vi "Read XML HW Configuration File_Extra Checks.vi"(8 "error in (no error)":errorcluster, 11 "Array In":T1[](array[typedef]) {"speed" items=["Auto", "Low", "High"]; "Labels"."scheduleBuildUnit" items=["Millisecond", "Microsecond"]}) -> (0 "error out":errorcluster, 3 "Array Out":T1[](array[typedef]) {"speed" items=["Auto", "Low", "High"]; "Labels"."scheduleBuildUnit" items=["Millisecond", "Microsecond"]})   [LabVIEW 2016]
doc: "This VI performs extra checks (to what is done via the XML Deserializer with the XSD)."
uses:
  Controls/Ballard_Channel.ctl
  Controls/Ballard_Label.ctl
  Controls/Ballard_Word.ctl
  Controls/ARINCParam.ctl
  Shared/Controls and Global/TransferType.ctl
  Controls/Channel_direction.ctl
  Controls/Channel Speed.ctl
  Shared/Ballard Arinc-429 Shared.lvlib
  Ballard Arinc-429 System Explorer.lvlib
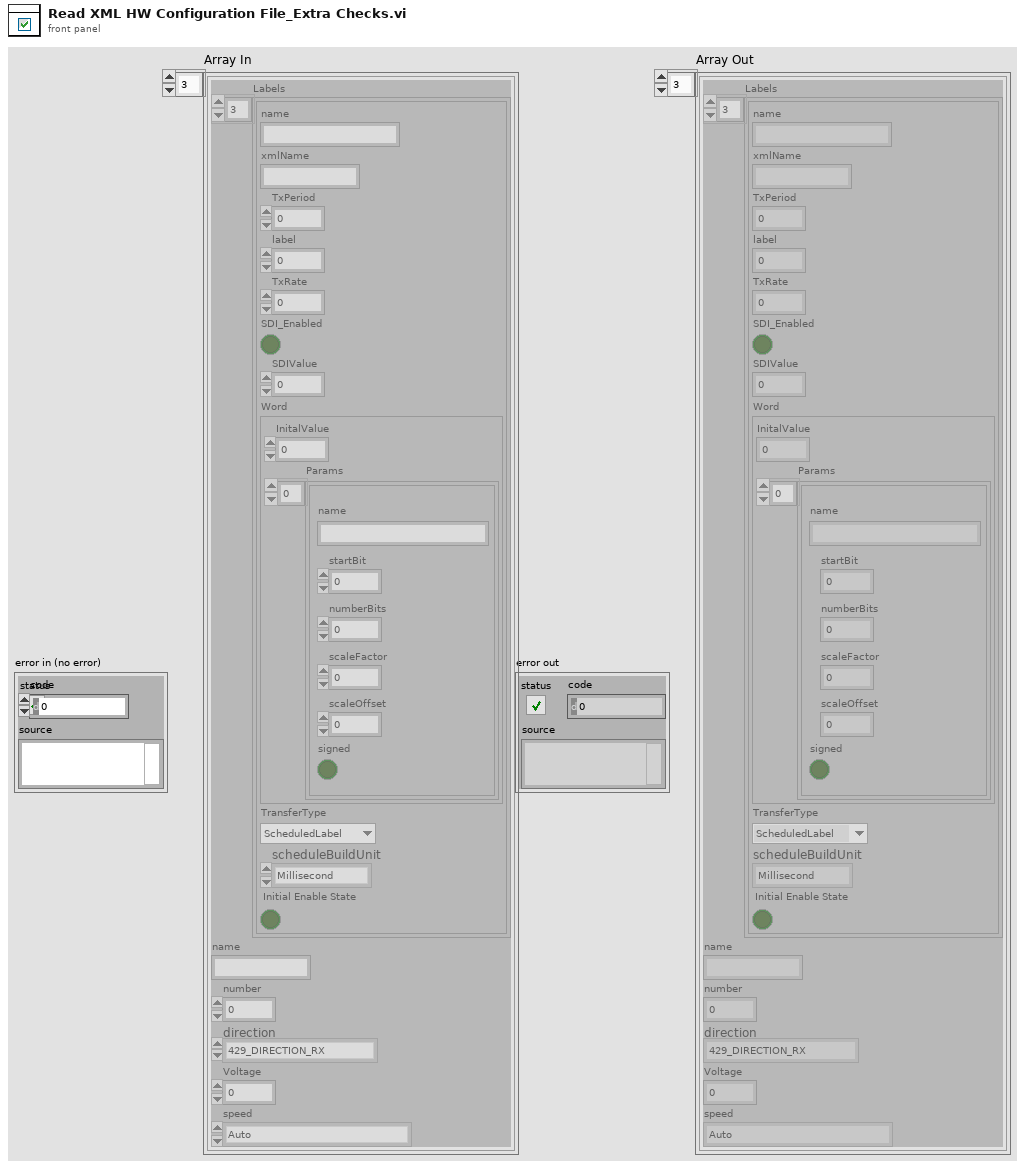
[diagram p1: front panel]
types:
  T1 = typedef "Ballard Arinc-429 System Explorer.lvlib/Ballard_Channel.ctl" = cluster{"Labels":T2[], "name":string, "number":u8, "direction":T6, "Voltage":dbl, "speed":T7}
  T2 = typedef "Ballard Arinc-429 System Explorer.lvlib/Ballard_Label.ctl" = cluster{"name":string, "xmlName":string, "TxPeriod":u32, "label":u32, "TxRate":dbl, "SDI_Enabled":bool, "SDIValue":u8, "Word":T3, "TransferType":T5, "scheduleBuildUnit":i32, "Initial Enable State":bool}
  T3 = typedef "Ballard Arinc-429 System Explorer.lvlib/Ballard_Word.ctl" = cluster{"InitalValue":u32, "Params":T4[]}
  T4 = typedef "Ballard Arinc-429 System Explorer.lvlib/ARINCParam.ctl" = cluster{"name":string, "startBit":i32, "numberBits":i32, "scaleFactor":dbl, "scaleOffset":dbl, "signed":bool}
  T5 = typedef "Ballard Arinc-429 Shared.lvlib/TransferType.ctl" = enum16{"ScheduledLabel", "Acyclic", "Block", "Strobe"}
  T6 = typedef "Ballard Arinc-429 System Explorer.lvlib/Channel_direction.ctl" = enum16{"429_DIRECTION_RX", "429_DIRECTION_TX"}
  T7 = typedef "Ballard Arinc-429 System Explorer.lvlib/Channel Speed.ctl" = i32
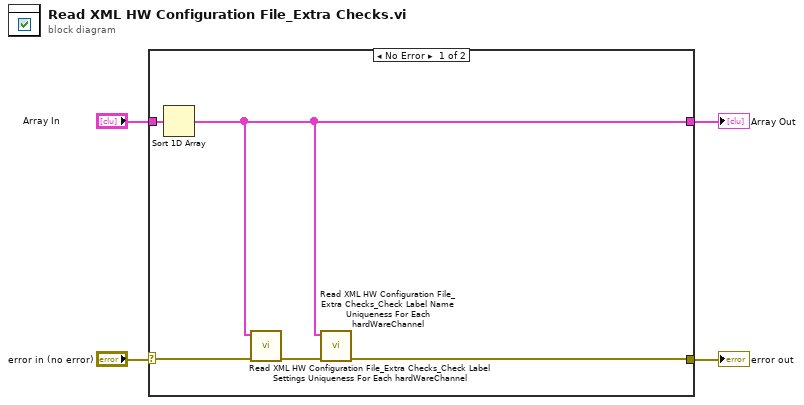
[diagram p0: block diagram]
diagram:
  n1 = case shown="No Error" "error in (no error)" {
    selector: "error in (no error)" -> [w8 w11]
    tunnel: [w5 w11] -> w3
    tunnel: "Array In" -> [w9 w10]
    tunnel: [w7 w10] -> w1
    frame No Error {
      n2 = Sort 1D Array(array=w9) -> (sorted array=w7:T1[])
      n3 = call "Read XML HW Configuration File_Extra Checks_Check Label Settings Uniqueness For Each hardWareChannel.vi"("error in (no error)"=w8, "Array In"=w7) -> ("error out"=w6:errorcluster)  [unwired: 9 in]
      n4 = call "Read XML HW Configuration File_Extra Checks_Check Label Name Uniqueness For Each hardWareChannel.vi"("error in (no error)"=w6, "Array In"=w7) -> ("error out"=w5:errorcluster)  [unwired: 9 in]
    }
    frame Error {
    }
  }
  "error out" <- w3
  "Array Out" <- w1
